vi "velocity_filter.vi"(10 "threshold":dbl, 11 "Array in":ext[](array[numeric])) -> (3 "index":i32[](array[numeric]))   [LabVIEW 2017]
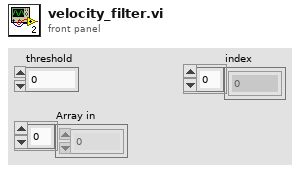
[diagram p1: front panel]
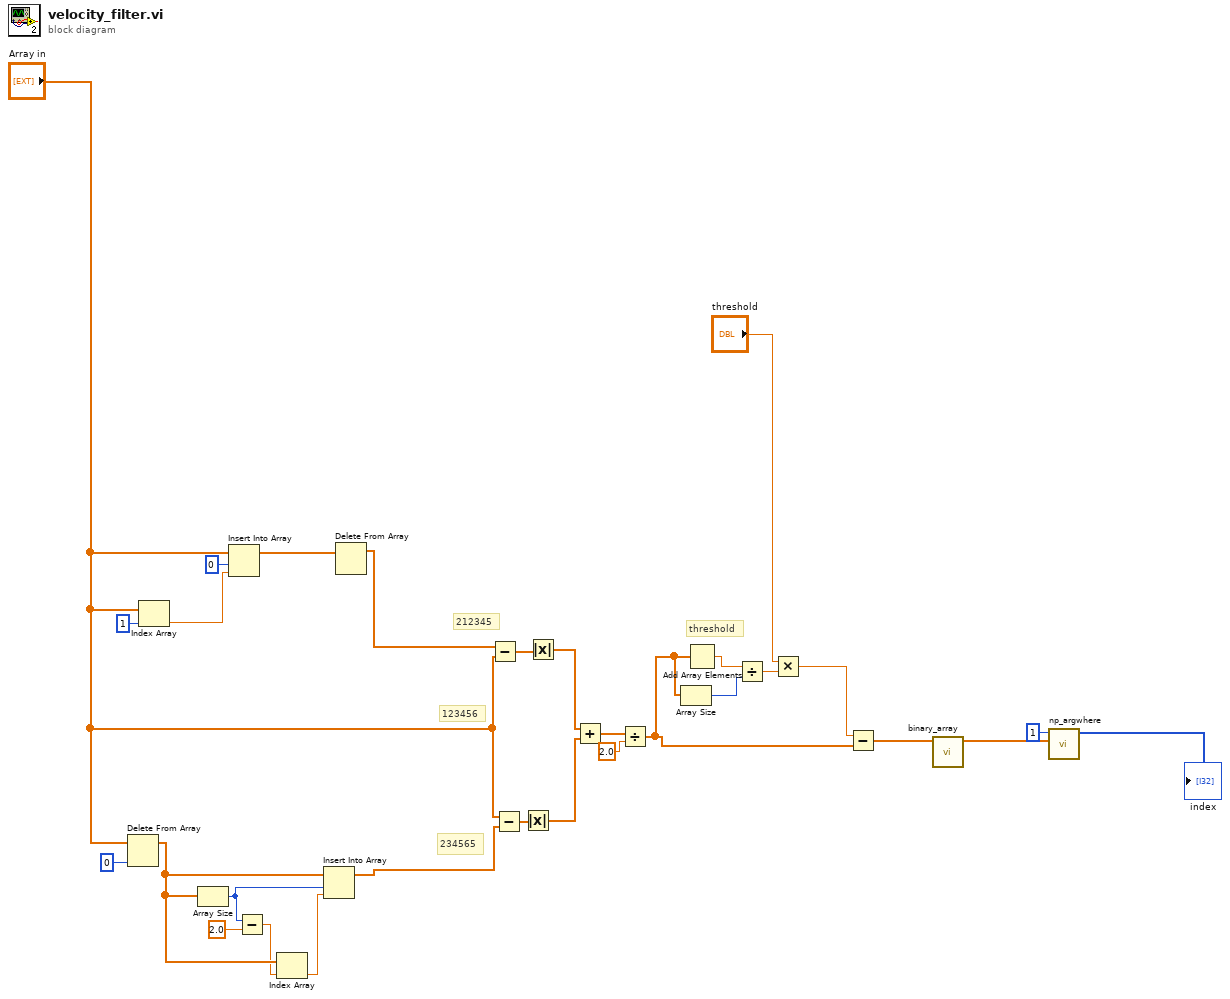
[diagram p0: block diagram]
diagram:
  # "threshold"
  # "234565"
  # "212345"
  # "123456"
  n1 = Delete From Array "Delete From Array"(array="Array in", index=0) -> (array with subset deleted=w9:ext[])  [unwired: 1 in, 1 out]
  n2 = Index Array "Index Array"(array="Array in", index=1) -> (element=w1:ext)
  n3 = Array Size(array=w9) -> (size(s)=w10:i32)
  n4 = Insert Into Array "Insert Into Array"(array="Array in", index=0, new element=w1) -> (w3:ext[])
  n5 = Subtract(x=w10, y=2.0) -> (x-y=w7:dbl)
  n6 = Index Array "Index Array"(array=w9, index=w7) -> (element=w8:ext)
  n7 = Insert Into Array "Insert Into Array"(array=w9, index=w10, new element=w8) -> (w13:ext[])
  n8 = Delete From Array "Delete From Array"(array=w3) -> (array with subset deleted=w11:ext[])  [unwired: 2 in, 1 out]
  n9 = Subtract(x=w11, y="Array in") -> (x-y=w14:ext[])
  n10 = Subtract(x="Array in", y=w13) -> (x-y=w15:ext[])
  n11 = Absolute Value(x=w15) -> (abs(x)=w17:ext[])
  n12 = Absolute Value(x=w14) -> (abs(x)=w16:ext[])
  n13 = Add(x=w16, y=w17) -> (x+y=w19:ext[])
  n14 = Divide(x=w19, y=2.0) -> (x/y=w24:ext[])
  n15 = Array Size(array=w24) -> (size(s)=w21:i32)
  n16 = Add Array Elements(numeric array=w24) -> (sum=w20:ext)
  n17 = Divide(x=w20, y=w21) -> (x/y=w22:ext)
  n18 = Multiply(x="threshold", y=w22) -> (x*y=w23:ext)
  n19 = Subtract(x=w23, y=w24) -> (x-y=w25:ext[])
  n20 = call "binary_array.vi"("Array"=w25) -> ("binary array"=w26:ext[])  [unwired: 10 in]
  n21 = call "np_argwhere.vi"("Array in"=w26, "value"=1) -> ("index"=→"index":i32[])  [unwired: 9 in]
